vi "ManipChangeState.vi"(3 "Instruction String":string) -> (0 "Error Out":errorcluster, 1 "Advance Trigger":bool)   [LabVIEW 2020]
doc: "This VI changes the robot's master state.\n\nParameters:\n1. state --> the robot's master state number"
uses:
  SafeParser_Integer.vi
  drivercommands.vi
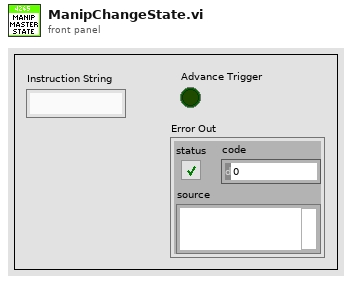
[diagram p1: front panel]
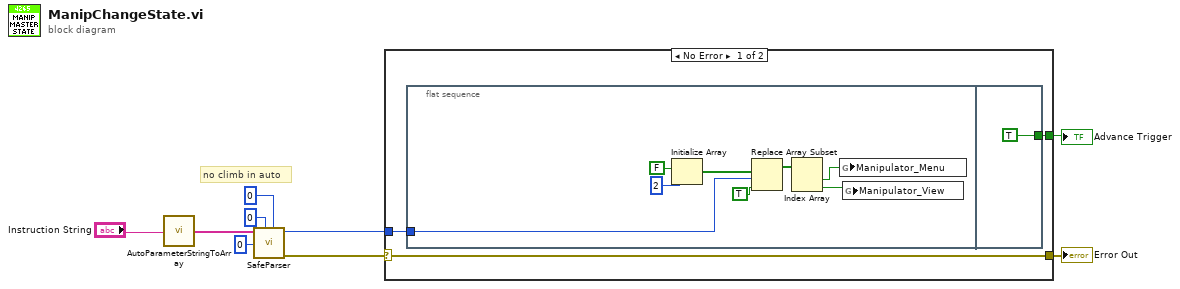
[diagram p0: block diagram]
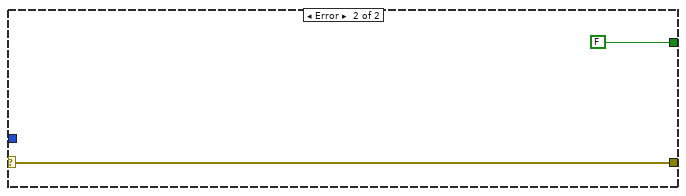
[diagram p2: hidden frame]
diagram:
  # "no climb in auto"
  n1 = call "AutoParameterStringToArray.vi"("Parameter String"="Instruction String") -> ("Parsed Parameters"=w5:string[])
  n2 = call-poly "SafeParser.vi"("Maximum"=0, "Minimum"=0, "Array Index"=0 ("Parameter Index"), "String Array"=w5) -> ("Error Out"=w7:errorcluster, "Typecast  Value"=w1:i32)  [unwired: 6 in]
  n3 = case shown="No Error" w7 {
    selector: w7 -> [w11 w23]
    tunnel: [w12 FALSE ("Advance Trigger")] -> w9
    tunnel: [w11 w23] -> w8
    tunnel: w1 -> [w10 _]
    frame No Error {
      n4 = flat-sequence {
        tunnel: w10 -> [w17]
        tunnel: [TRUE ("Advance Trigger")] -> w12
        frame #0 {
          n5 = Initialize Array(FALSE, 2 ("dimension size")) -> (w18:bool[])
          n6 = Replace Array Subset(array=w18, new element=TRUE ("new element/subarray"), index=w17) -> (w15:bool[])
          n7 = Index Array(array=w15) -> (element #1=w14:bool, element #2=w13:bool)  [unwired: 2 in]
          n8 = global write "drivercommands.vi" "Manipulator_Menu"(w14) -> ()
          n9 = global write "drivercommands.vi" "Manipulator_View"(w13) -> ()
        }
        frame #1 {
        }
      }
    }
    frame Error {
    }
  }
  "Advance Trigger" <- w9
  "Error Out" <- w8
